vi "CRYCurve to Table.vi"(8 "y precision":u8=2, 9 "Margin":bool, 10 "x precision":u8=2, 11 "Limit curve In":cluster{"Numeric":dbl, "Numeric 2":dbl}[](array[cluster]) {"Numeric 2" format="%#.8p"; "Numeric" format="%#.8p"}) -> (0 "Single value":dbl format="%.1p", 3 "Limit Table":string[][](array[string]))   [LabVIEW 2013]
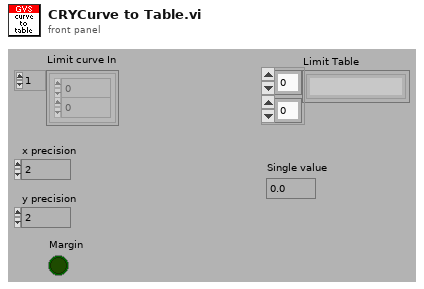
[diagram p1: front panel]
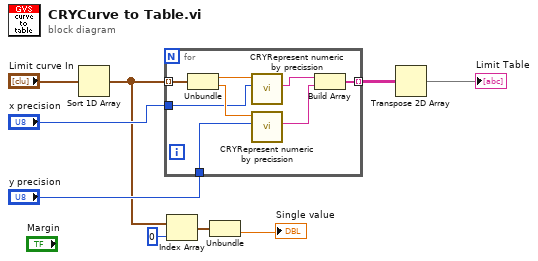
[diagram p0: block diagram]
diagram:
  n1 = Sort 1D Array(array="Limit curve In") -> (sorted array=w2:cluster{"Numeric":dbl, "Numeric 2":dbl}[])
  n2 = for {
    tunnel: w2 -> [w17] mode=indexing
    tunnel: [w16] -> w9 mode=indexing
    tunnel: "x precision" -> [w13]
    tunnel: "y precision" -> [w12]
    n3 = Unbundle(w17) -> ("Numeric"=w15:dbl, "Numeric 2"=w14:dbl)
    n4 = call "CRYRepresent numeric by precission.vi"("Pprecision"=w13, "Numeric In"=w15) -> ("output string"=w11:string)  [unwired: 7 in, 2 out]
    n5 = call "CRYRepresent numeric by precission.vi"("Pprecision"=w12, "Numeric In"=w14) -> ("output string"=w10:string)  [unwired: 7 in, 2 out]
    n6 = Build Array(w11, w10) -> (w16:string[])
  }
  n7 = Index Array(array=w2, index=0 ("Index")) -> (element=w7:cluster{"Numeric":dbl, "Numeric 2":dbl})
  n8 = Unbundle(w7) -> ("Numeric 2"=→"Single value":dbl)  [unwired: 1 out]
  n9 = Transpose 2D Array(2D array=w9) -> (transposed array=→"Limit Table":string[][])
